vi "Test IPS120 comms.vi"(8 "Error In":errorcluster, 9 "Command 2":string="J1.5\r", 10 "Command 1":string="A1\r", 11 "VISA resource name":refnum<visa-resource-name>) -> (0 "Error Out":errorcluster, 3 "VISA resource name out":refnum<visa-resource-name>)   [LabVIEW 2018]
uses:
  IPS120.lvclass
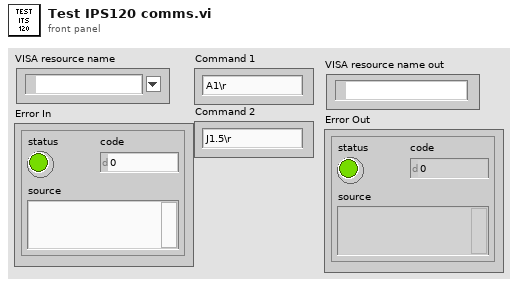
[diagram p1: front panel]
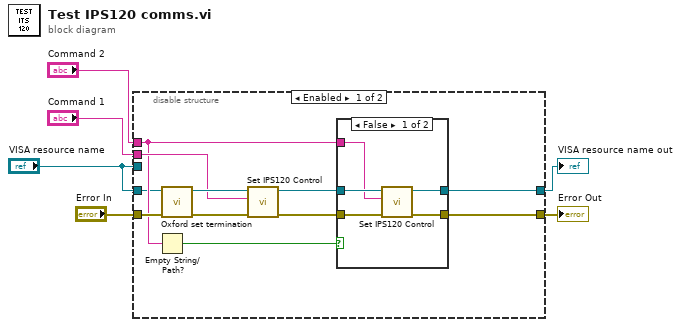
[diagram p0: block diagram]
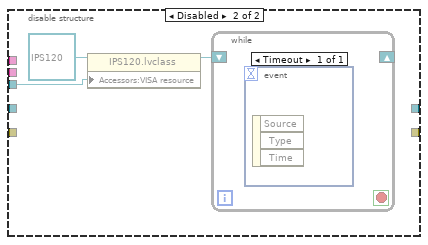
[diagram p3: hidden frame]
diagram:
  n1 = disable-structure shown="Enabled" {
    disable-tunnel: "Error In" -> [w15 _]
    disable-tunnel: "Command 1" -> [w14 _]
    disable-tunnel: [w11 _] -> w4
    disable-tunnel: [w10 _] -> w3
    disable-tunnel: "Command 2" -> [w9 _]
    disable-tunnel: "VISA resource name" -> [w7 _]
    disable-tunnel: "VISA resource name" -> [_ w25]
    frame Enabled {
      n2 = Empty String/Path?(string/path=w9) -> (empty?=w8:bool)
      n3 = call "Oxford set termination.vi"("error in (no error)"=w15, "VISA resource name"=w7) -> ("error out"=w17:errorcluster, "VISA resource name out"=w16:refnum<visa-resource-name>)  [unwired: 8 in]
      n4 = call "Set IPS120 Control.vi"("Error In"=w17, "Command string"=w14, "VISA resource name"=w16) -> ("Error Out"=w13:errorcluster, "VISA resource name out"=w12:refnum<visa-resource-name>)  [unwired: 7 in]
      n5 = case shown="False" w8 {
        tunnel: w13 -> [w22 w23]
        tunnel: w12 -> [w21 w24]
        tunnel: [w20 w24] -> w11
        tunnel: w9 -> [w19 _]
        tunnel: [w18 w23] -> w10
        frame False {
          n6 = call "Set IPS120 Control.vi"("Error In"=w22, "Command string"=w19, "VISA resource name"=w21) -> ("Error Out"=w18:errorcluster, "VISA resource name out"=w20:refnum<visa-resource-name>)  [unwired: 7 in]
        }
        frame True {
        }
      }
    }
    frame Disabled {
      n7 = property class="IPS120.lvclass"(reference=refnum<class "IPS120.lvclass"> refnum ("IPS120.lvclass"), "Accessors:VISA resource"=w25) -> (reference out=w27:refnum<class "IPS120.lvclass">)  [unwired: 1 in, 1 out]
      n8 = while {
        shift-right: _ -> [_]
        shift-left: w27 -> [_]
        stop <- _ stop-if-true
        n9 = event shown="[0] Timeout" {
          selector: _ -> [_]
          dyn-events: _ -> [_]
          timeout: _ -> [_]
          event Timeout {
            n10 = event-data() -> ()  [unwired: 1 in, 3 out]
          }
        }
      }
    }
  }
  "VISA resource name out" <- w4
  "Error Out" <- w3
